vi "选择奶茶目录.vi"(8 "error in (no error)":errorcluster caption="错误输入（无错误）", 10 "选择目录":dbl, 11 "奶茶 输入":refnum<class "奶茶.lvclass">) -> (0 "error out":errorcluster caption="错误输出", 2 "特定类引用":refnum<class "奶茶.lvclass">, 3 "奶茶 输出":refnum<class "奶茶.lvclass">)   [LabVIEW 2016, in "奶茶.lvclass"]
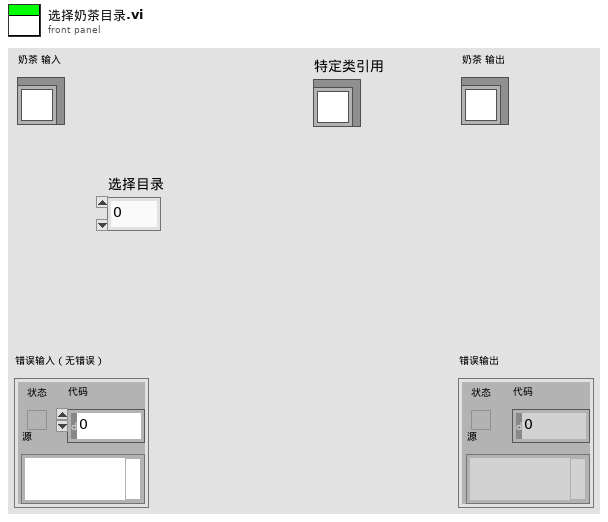
[diagram p1: front panel]
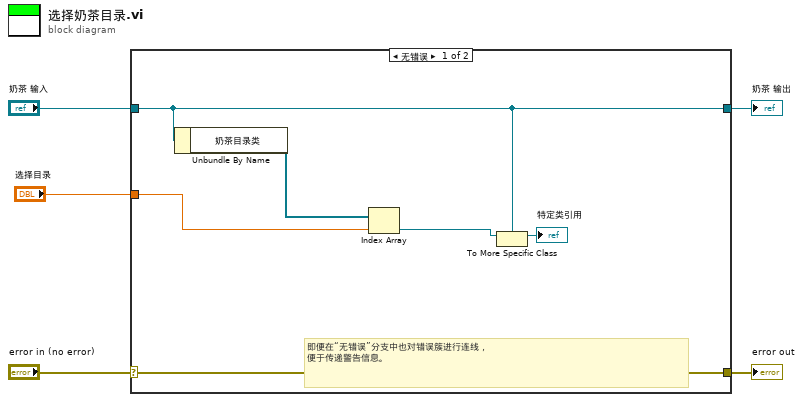
[diagram p0: block diagram]
diagram:
  n1 = case shown="无错误" "error in (no error)" {
    selector: "error in (no error)" -> [w11 w13]
    tunnel: [w11 w13] -> w4
    tunnel: [w7 w12] -> w2
    tunnel: "奶茶 输入" -> [w7 w12]
    tunnel: "选择目录" -> [w9 _]
    frame No Error {
      # "即便在“无错误”分支中也对错误簇进行连线，\n便于传递警告信息。"
      n2 = Unbundle By Name(w7) -> ("奶茶目录类"=w10:refnum<class>[])
      n3 = Index Array(array=w10, index=w9) -> (element=w8:refnum<class>)
      n4 = To More Specific Class(target class=w7, reference=w8) -> (specific class reference=→"特定类引用":refnum<class "奶茶.lvclass">)  [unwired: 1 in, 1 out]
    }
    frame Error {
    }
  }
  "error out" <- w4
  "奶茶 输出" <- w2
